vi "DSF.Engine.Plugin.Tx.Inline.Start.vi"(8 "error in (no error)":errorcluster, 11 "Plugin in":refnum<class "DSF.Engine.Plugin.lvclass">) -> (0 "error out":errorcluster, 3 "Plugin out":refnum<class "DSF.Engine.Plugin.lvclass">)   [LabVIEW 2017, in "DSF.Engine.lvlib" / "DSF.Engine.Plugin.lvclass"]
uses:
  DSF.Engine.Plugin.lvclass
  DSF.Engine.Plugin.lvclass/DSF.Engine.Plugin.ctl
  Transfer/DSF.Engine.Transfer Group.lvclass/DSF.Engine.Transfer Group.ctl
  Timing/DSF.Engine.Timing.lvclass/DSF.Engine.Timing.ctl
  Transfer/DSF.Engine.Transfer Group.Increment Iteration.vi
  Transfer/DSF.Engine.Transfer Group.Get Timing.vi
  Transfer/DSF.Engine.Transfer Group.Set Timing.vi
  Timing/DSF.Engine.Timing.Iteration.Increment.vi
  Timing/DSF.Engine.Timing.Get Iteration.vi
  Timing/DSF.Engine.Timing.Set Iteration.vi
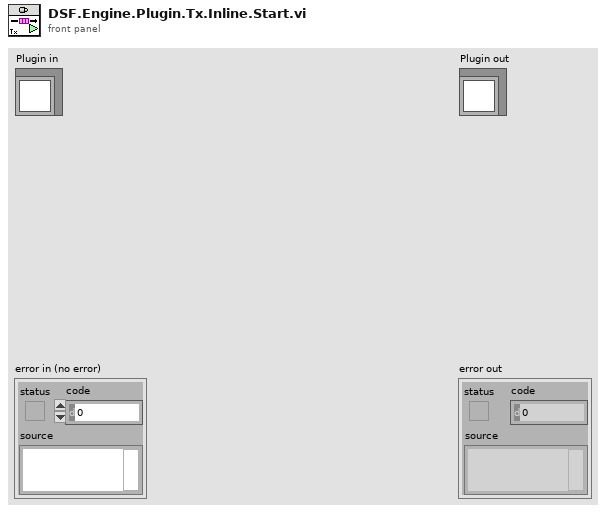
[diagram p1: front panel]
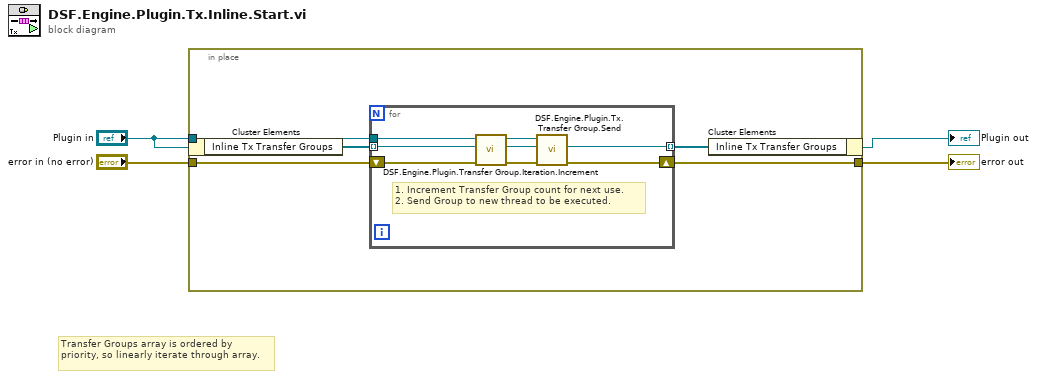
[diagram p0: block diagram]
diagram:
  # "Transfer Groups array is ordered by priority, so linearly iterate through array."
  n1 = in-place {
    in-place-border: "error in (no error)" -> [w9]
    in-place-border: [w8] -> w3
    in-place-border: "Plugin in" -> [w6]
    n2 = in-place-cluster #1("Plugin in") -> ("Inline Tx Transfer Groups"=w7:refnum<class "DSF.Engine.Transfer Group.lvclass">[])
    n3 = for {
      tunnel: w7 -> [w12] mode=indexing
      shift-right: [w17] -> w8
      shift-left: w9 -> [w10]
      tunnel: [w16] -> w5 mode=indexing
      tunnel: w6 -> [w11]
      # "1. Increment Transfer Group count for next use.\n2. Send Group to new thread to be executed."
      n4 = call "DSF.Engine.Plugin.Transfer Group.Iteration.Increment.vi"("error in (no error)"=w10, "Transfer Group in"=w12, "Plugin in"=w11) -> ("error out"=w14:errorcluster, "Transfer Group out"=w13:refnum<class "DSF.Engine.Transfer Group.lvclass">, "Plugin out"=w15:refnum<class "DSF.Engine.Plugin.lvclass">)  [unwired: 6 in]
      n5 = call "DSF.Engine.Plugin.Tx.Transfer Group.Send.vi"("error in (no error)"=w14, "Transfer Group in"=w13, "Plugin in"=w15) -> ("error out"=w17:errorcluster, "Transfer Group out"=w16:refnum<class "DSF.Engine.Transfer Group.lvclass">)  [unwired: 6 in, 1 out]
    }
    n6 = in-place-cluster #1("Inline Tx Transfer Groups"=w5) -> (→"Plugin out":refnum<class "DSF.Engine.Plugin.lvclass">)
  }
  "error out" <- w3
